vi "RampInFlow.vi"(0 "object in":refnum<class "CetoniPump.lvclass">, 2 "Ramp In Settings":T1, 5 "error in (no error)":errorcluster) -> (14 "object out":refnum<class "CetoniPump.lvclass">, 16 "Target Level Reached":bool, 17 "Pump Status out":T2(array[cluster]), 19 "error out":errorcluster)   [LabVIEW 2021, in "CetoniPump.lvclass"]
uses:
  CetoniPump.lvclass
  CetoniPump.lvclass/CetoniPump.ctl
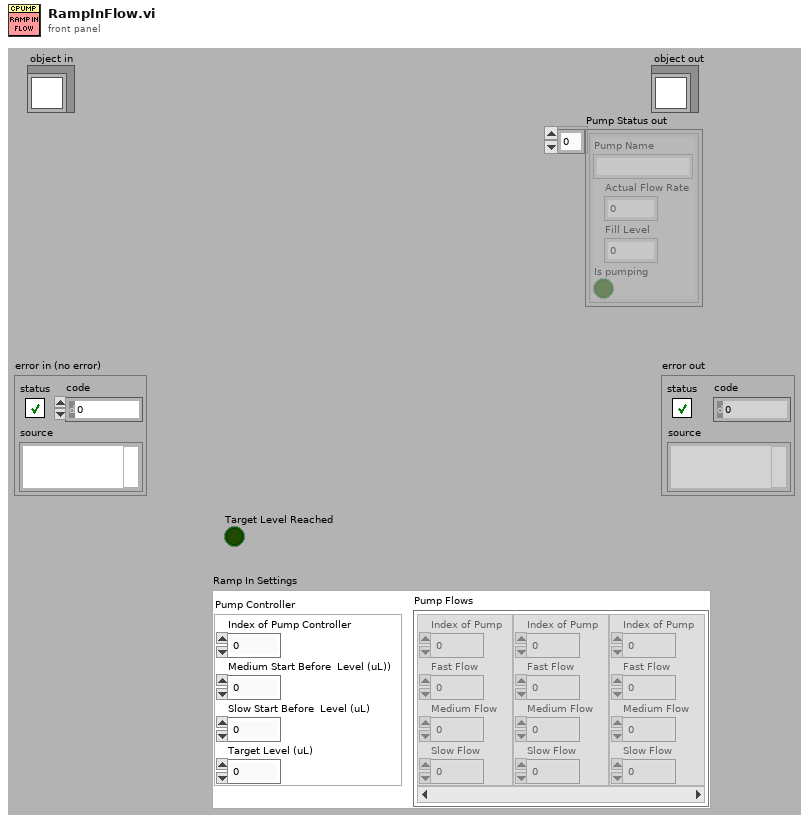
[diagram p1: front panel]
types:
  T1 = cluster{"Pump Controller":cluster{"Index of Pump Controller":u8, "Medium Start Before  Level (uL))":dbl, "Slow Start Before  Level (uL)":dbl, "Target Level (uL)":dbl}, "Pump Flows":cluster{"Index of Pump":u8, "Fast Flow":dbl, "Medium Flow":dbl, "Slow Flow":dbl}[]}
  T2 = cluster{"Pump Name":string, "Actual Flow Rate":dbl, "Fill Level":dbl, "Is pumping":bool}[]
  T3 = cluster{"Index of Pump":u8, "Fast Flow":dbl, "Medium Flow":dbl, "Slow Flow":dbl}[]
  T4 = cluster{"Pump Name":string, "Actual Flow Rate":dbl, "Fill Level":dbl, "Is pumping":bool}
  T5 = cluster{"Pump Handle":i64, "Pump Name":string, "Maximum Volume":dbl, "Maximum Flow Rate":dbl, "Flow Rate":dbl, "Target Level":dbl}[]
  T6 = cluster{"Pump Handle":i64, "Pump Name":string, "Maximum Volume":dbl, "Maximum Flow Rate":dbl, "Flow Rate":dbl, "Target Level":dbl}
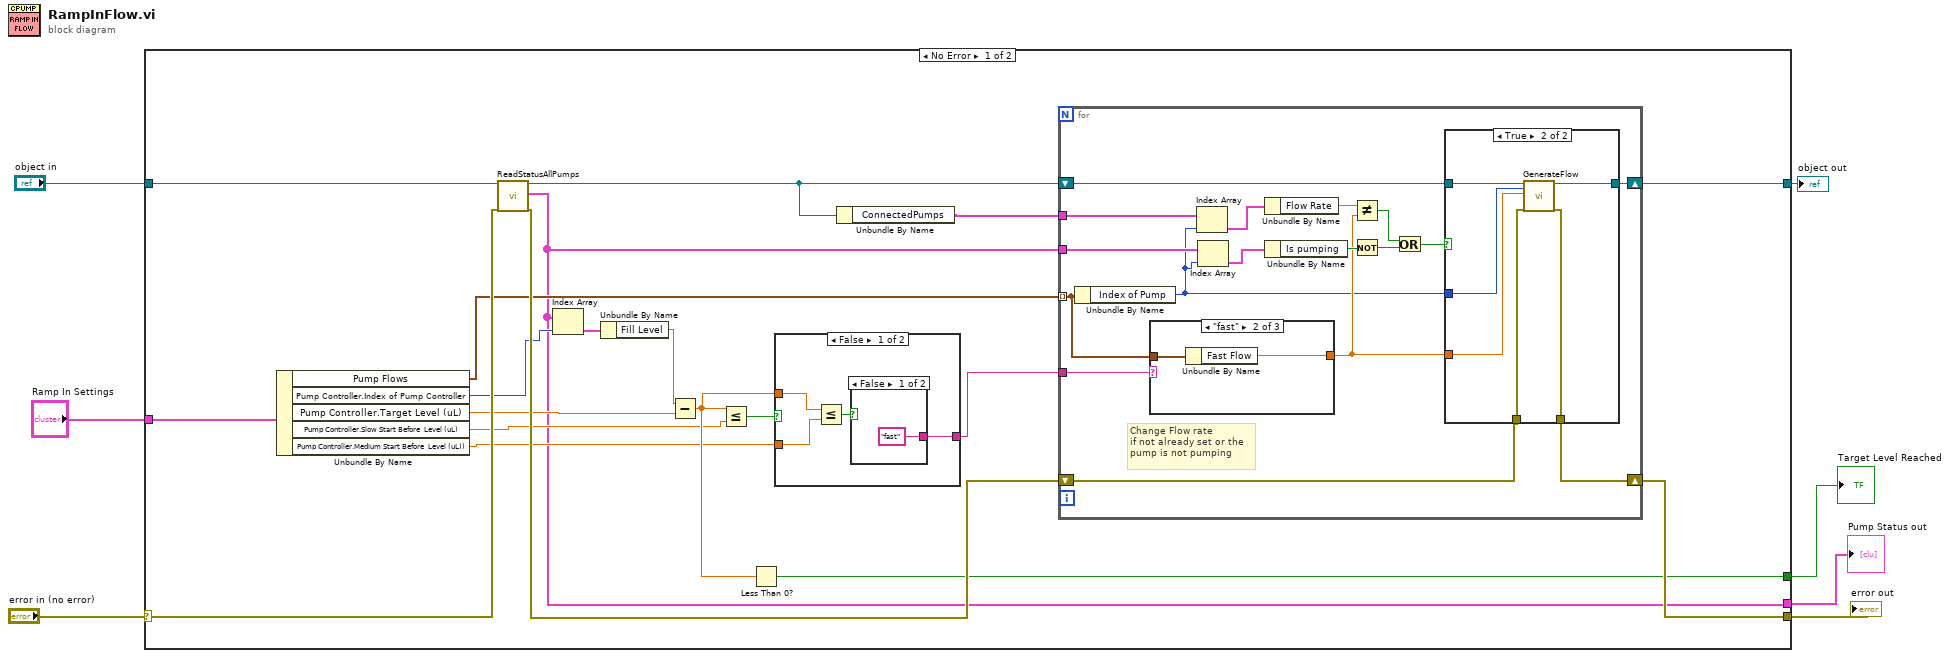
[diagram p0: block diagram]
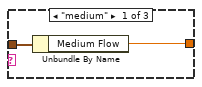
[diagram p2: hidden frame]
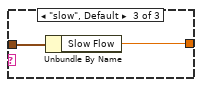
[diagram p3: hidden frame]
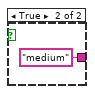
[diagram p5: hidden frame]
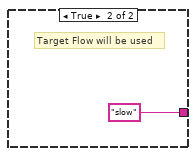
[diagram p6: hidden frame]
diagram:
  n1 = case shown="No Error" "error in (no error)" {
    selector: "error in (no error)" -> [w27 w67]
    tunnel: [w22 w67] -> w6
    tunnel: [w24 w66] -> w4
    tunnel: "object in" -> [w25 w66]
    tunnel: [w20 _] -> w3
    tunnel: [w9 _] -> w2
    tunnel: "Ramp In Settings" -> [w12 _]
    frame No Error {
      n2 = Unbundle By Name(w12) -> ("Pump Flows"=w11:T3, "Pump Controller.Index of Pump Controller"=w16:u8, "Pump Controller.Target Level (uL)"=w15:dbl, "Pump Controller.Slow Start Before  Level (uL)"=w14:dbl, "Pump Controller.Medium Start Before  Level (uL))"=w13:dbl)
      n3 = call-dynamic "ReadStatusAllPumps.vi"("object in"=w25, "error in (no error)"=w27) -> ("object out"=w17:refnum<class "CetoniPump.lvclass">, "Array"=w9:T2, "error out"=w23:errorcluster)  [unwired: 15 in]
      n4 = Index Array(array=w9, index=w16) -> (element=w19:T4)
      n5 = Unbundle By Name(w19) -> ("Fill Level"=w18:dbl)
      n6 = Subtract(x=w18, y=w15) -> (x-y=w21:dbl)
      n7 = Less Or Equal?(x=w21, y=w14) -> (x <= y?=w26:bool)
      n8 = Less Than 0?(x=w21) -> (x < 0?=w20:bool)
      n9 = case shown="False" w26 {
        tunnel: w13 -> [w62 _]
        tunnel: w21 -> [w61 _]
        tunnel: [w59 "slow"] -> w8
        frame False {
          n10 = Less Or Equal?(x=w61, y=w62) -> (x <= y?=w60:bool)
          n11 = case shown="False" w60 {
            tunnel: ["fast" "medium"] -> w59
            frame False {
            }
            frame True {
            }
          }
        }
        frame True {
          # "Target Flow will be used"
        }
      }
      n12 = Unbundle By Name(w17) -> ("ConnectedPumps"=w10:T5)
      n13 = for {
        shift-right: [w42] -> w24
        shift-left: w17 -> [w43]
        shift-right: [w40] -> w22
        shift-left: w23 -> [w41]
        tunnel: w11 -> [w32] mode=indexing
        tunnel: w10 -> [w37]
        tunnel: w9 -> [w30]
        tunnel: w8 -> [w33]
        # "Change Flow rate \nif not already set or the \npump is not pumping"
        n14 = Unbundle By Name(w32) -> ("Index of Pump"=w29:u8)
        n15 = case shown="\"fast\"" w33 {
          tunnel: w32 -> [w46 w48 w50]
          tunnel: [w45 w47 w49] -> w31
          frame "medium" {
            n16 = Unbundle By Name(w46) -> ("Medium Flow"=w45:dbl)
          }
          frame "fast" {
            n17 = Unbundle By Name(w48) -> ("Fast Flow"=w47:dbl)
          }
          frame "slow", Default {
            n18 = Unbundle By Name(w50) -> ("Slow Flow"=w49:dbl)
          }
        }
        n19 = Index Array(array=w37, index=w29) -> (element=w36:T6)
        n20 = Index Array(array=w30, index=w29) -> (element=w28:T4)
        n21 = Unbundle By Name(w36) -> ("Flow Rate"=w44:dbl)
        n22 = Unbundle By Name(w28) -> ("Is pumping"=w39:bool)
        n23 = Not Equal?(x=w44, y=w31) -> (x != y?=w35:bool)
        n24 = Not(x=w39) -> (.not. x?=w34:bool)
        n25 = Or(x=w35, y=w34) -> (x .or. y?=w38:bool)
        n26 = case shown="True" w38 {
          tunnel: w43 -> [w52 w58]
          tunnel: [w52 w57] -> w42
          tunnel: w41 -> [w51 w56]
          tunnel: [w51 w55] -> w40
          tunnel: w29 -> [_ w54]
          tunnel: w31 -> [_ w53]
          frame False {
          }
          frame True {
            n27 = call-dynamic "GenerateFlow.vi"("object in"=w58, "index"=w54, "Flow Rate"=w53, "error in (no error)"=w56) -> ("object out"=w57:refnum<class "CetoniPump.lvclass">, "error out"=w55:errorcluster)  [unwired: 14 in]
          }
        }
      }
    }
    frame Error {
    }
  }
  "error out" <- w6
  "object out" <- w4
  "Target Level Reached" <- w3
  "Pump Status out" <- w2
